vi "GoBack.vi"(8 "error in (no error)":errorcluster, 11 "SMO.Activity in":refnum<class "SMO.Activity.lvclass">) -> (0 "error out":errorcluster, 3 "SMO.Activity out":refnum<class "SMO.Activity.lvclass">)   [LabVIEW 2015, in "SMO.Activity.lvclass"]
uses:
  SMO.Activity.lvclass
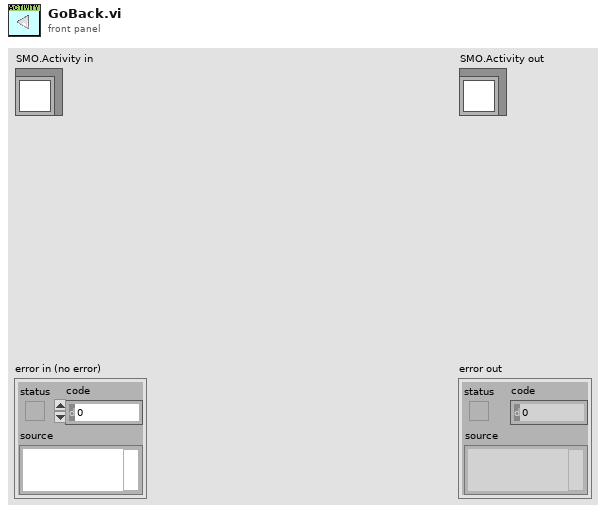
[diagram p1: front panel]
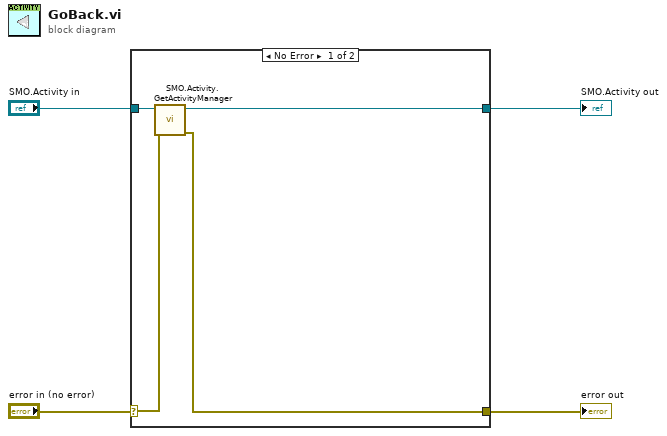
[diagram p0: block diagram]
diagram:
  n1 = case shown="No Error" "error in (no error)" {
    selector: "error in (no error)" -> [w6 w10]
    tunnel: [w5 w10] -> w3
    tunnel: [w7 w9] -> w1
    tunnel: "SMO.Activity in" -> [w8 w9]
    frame No Error {
      n2 = call "SMO.Activity.GetActivityManager.vi"("error in (no error)"=w6, "SMO.Activity"=w8) -> ("error out"=w5:errorcluster, "SMO.Activity out"=w7:refnum<class "SMO.Activity.lvclass">)  [unwired: 7 in, 1 out]
    }
    frame Error {
    }
  }
  "error out" <- w3
  "SMO.Activity out" <- w1
